vi "OPA.GetShutterState.vi"(8 "error in (no error)":errorcluster, 11 "OPA.OrpheusHP in":refnum<class "OPA.OrpheusHP.lvclass">) -> (0 "error out":errorcluster, 2 "Shutter State":bool, 3 "OPA.OrpheusHP out":refnum<class "OPA.OrpheusHP.lvclass">)   [LabVIEW 2019, in "OPA.OrpheusHP.lvclass"]
uses:
  OPA.OrpheusHP.lvclass
  E:/UPWORK/Laser Tool/Topas4PublicAPI/NET_SDK/Topas4Lib.dll
  Topas4PublicAPI/NET_SDK/Topas4Lib.dll
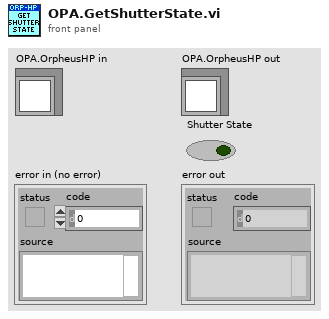
[diagram p1: front panel]
types:
  T1 = typedef "OPA.OrpheusHP.lvclass/Resource--Cluster.ctl" = cluster{"TopasDevice":refnum<k24>, "WavelengthService":refnum<k24>, "ShutterService":refnum<k24>}
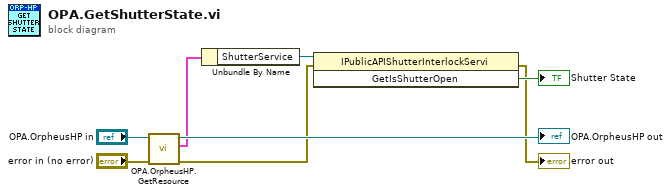
[diagram p0: block diagram]
diagram:
  n1 = call "OPA.OrpheusHP.GetResource.vi"("error in (no error)"="error in (no error)", "OPA.OrpheusHP in"="OPA.OrpheusHP in") -> ("error out"=w2:errorcluster, "Resource"=w5:T1, "OPA.OrpheusHP out"=→"OPA.OrpheusHP out":refnum<class "OPA.OrpheusHP.lvclass">)  [unwired: 7 in]
  n2 = Unbundle By Name(w5) -> ("ShutterService"=w4:refnum<k24>)
  n3 = invoke class="IPublicAPIShutterInterlockServi" method="GetIsShutterOpen"(reference=w4, error in=w2) -> (error out=→"error out":errorcluster, "GetIsShutterOpen"=→"Shutter State":bool)  [unwired: 1 in, 1 out]
